vi "Wait for End-of-File.vi"(5 "Username":string, 6 "Password":string, 7 "Address":string, 8 "Error In":errorcluster) -> (0 "Error Out":errorcluster)   [LabVIEW 2018, in "Tests.lvlib" / "Channel.lvlib"]
uses:
  Channel.lvlib
  <vilib>/addons/_JKI Toolkits/Caraya/classes/Test/Test.lvclass
  <vilib>/addons/_JKI Toolkits/Caraya/classes/Assert/Assert.lvclass
  src/Toolkit/API/Channel/Channel.lvclass
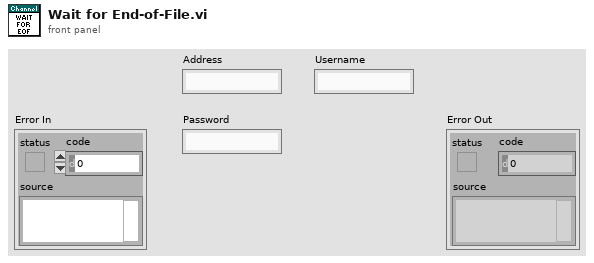
[diagram p1: front panel]
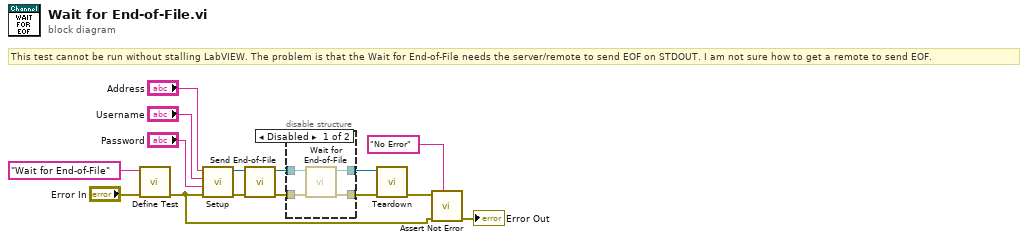
[diagram p0: block diagram]
diagram:
  # "This test cannot be run without stalling LabVIEW. The problem is that the Wait for End-of-File needs the server/remote to send EOF on STDOUT. I am not sure how to get a remote to send EOF."
  n1 = call <vilib>:"Define Test.vi"("error in (no error)"="Error In", "Label (VI Title)"="Wait for End-of-File") -> ("error out"=w12:errorcluster)  [unwired: 9 in]
  n2 = call "Setup.vi"("Error In"=w12, "Password"="Password", "Username"="Username", "Address"="Address") -> ("Error Out"=w5:errorcluster, "Channel"=w6:refnum<class "Channel.lvclass">)  [unwired: 6 in]
  n3 = call "Send End-of-File.vi"("Error In"=w5, "Channel In"=w6) -> ("Error Out"=w3:errorcluster, "Channel Out"=w4:refnum<class "Channel.lvclass">)  [unwired: 8 in]
  n4 = disable-structure shown="Disabled" {
    disable-tunnel: w4 -> [w19 w21]
    disable-tunnel: w3 -> [w18 w20]
    disable-tunnel: [w17 w20] -> w2
    disable-tunnel: [w16 w21] -> w1
    frame Disabled {
      n5 = call "Wait for End-of-File.vi"("Error In"=w18, "Channel In"=w19) -> ("Error Out"=w17:errorcluster, "Channel Out"=w16:refnum<class "Channel.lvclass">)  [unwired: 8 in]
    }
    frame Enabled {
    }
  }
  n6 = call "Teardown.vi"("Error In"=w2, "Channel"=w1) -> ("Error Out"=w8:errorcluster)  [unwired: 9 in]
  n7 = call <vilib>:"Assert Not Error.vi"("Label"="No Error", "error in (no error)"=w12, "Not Error?"=w8) -> ("error out"=→"Error Out":errorcluster)  [unwired: 8 in]
